vi "Startup.vi"(6 "LabVIEW Web Service":refnum<class "Web Service.lvclass">) -> ()   [LabVIEW 2014]
uses:
  <vilib>/wsapi/Web Service.lvclass
  DataManager/StateStore/Controls/DataFunction.ctl
panel:
  out "Array":cluster{"uuid":string, "int":i32}[](array[cluster])
  out "data out 2":string
  out "timing get SW 2":u32
  out "timing post SW 2":u32
  out "timing get 3":u32
  out "sum 2":i32
  out "timing post 2":u32
  out "timing get SW":u32
  out "timing post SW":u32
  out "timing post 1":u32
  out "data out":string
  out "service stopping?":bool
  out "timing get 2":u32
  out "sum":i32
  # "Use the web service input terminal to call the VIs on the Service subpalette of the Web Services palette. Do not remove it from the connector pane unless you don't need access to the palette."
  # "Any additional terminals added to the connector pane of a startup VI will be ignored."
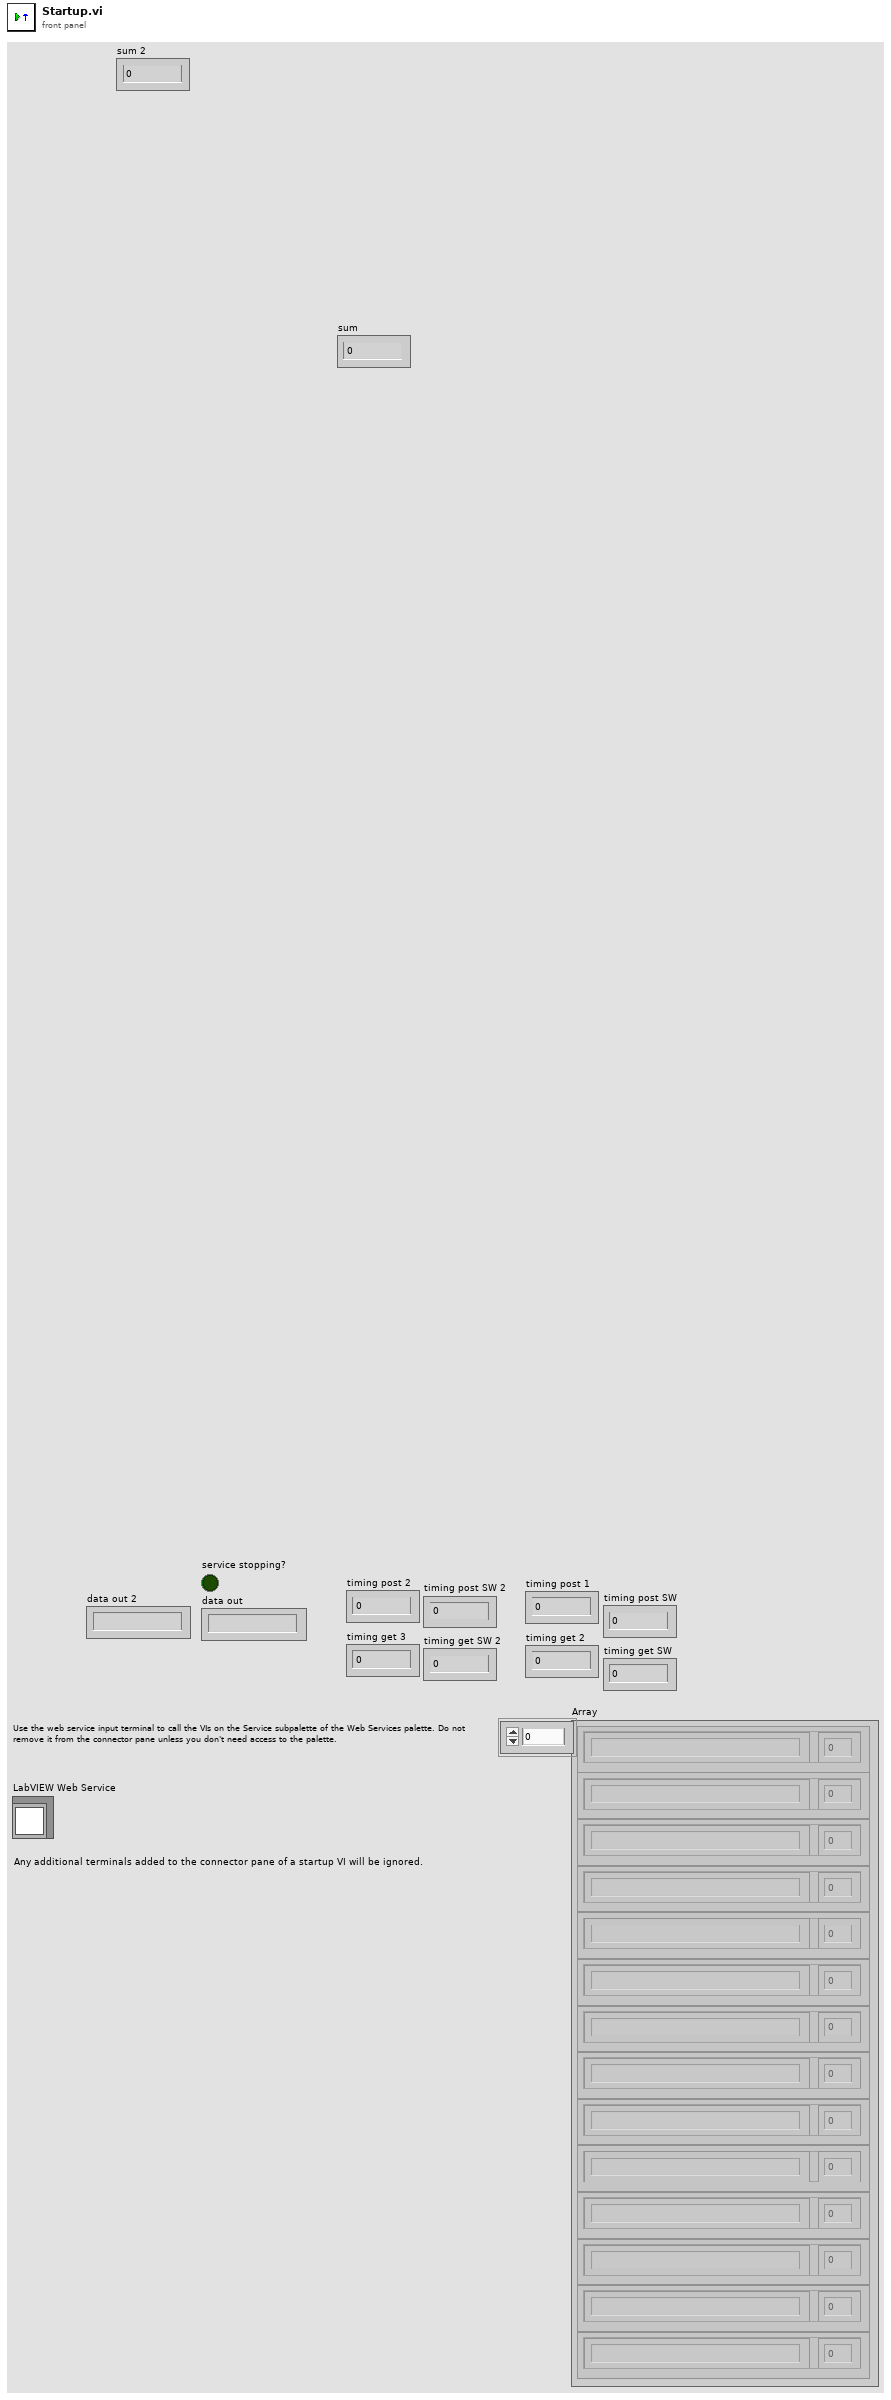
[diagram p1: front panel]
types:
  T1 = typedef "DataFunction.ctl" = enum16{"Initialise", "Release", "Get Data", "Set Data", "Preview Data"}
  T2 = enum16{"Standard", "Buffered", "CRLF", "Immediate"}
  T3 = cluster{"uuid":string, "int":i32, "posit_array":cluster{"x":dbl, "y":dbl, "z":dbl}[]}[]
  T4 = cluster{"0":string, "1":dbl, "2":dbl, "3":dbl, "4":dbl, "5":string, "6":string, "7":string}
  T5 = cluster{"switch_posit":cluster{"x":dbl, "y":dbl, "z":dbl}, "manual":bool}
  T6 = typedef "CData Core Control.ctl" = cluster{"train_data_array":cluster{"uuid":string, "int":i32, "posit_array":cluster{"x":dbl, "y":dbl, "z":dbl}[]}[], "train_control_array":cluster{"uuid":string, "throttle":dbl, "brake":dbl, "horn":dbl, "wait":dbl, "name":string, "mode":string, "dest":string}[], "switch_data_array":cluster{"switch_posit":cluster{"x":dbl, "y":dbl, "z":dbl}, "manual":bool}[], "switch_control_array":cluster{"switch_posit":cluster{"x":dbl, "y":dbl, "z":dbl}, "switch":bool, "invert":bool, "wait":dbl}[]}
  T7 = cluster{"uuid":string, "throttle":dbl, "brake":dbl, "horn":dbl, "wait":dbl, "name":string, "mode":string, "dest":string}[]
  T8 = cluster{"switch_posit":cluster{"x":dbl, "y":dbl, "z":dbl}, "manual":bool}[]
  T9 = cluster{"switch_posit":cluster{"x":dbl, "y":dbl, "z":dbl}, "switch":bool, "invert":bool, "wait":dbl}
  T10 = cluster{"switch_posit":cluster{"x":dbl, "y":dbl, "z":dbl}, "switch":bool, "invert":bool, "wait":dbl}[]
  T11 = cluster{"switch_posit":cluster{"x":dbl, "y":dbl, "z":dbl}, "switch":bool}
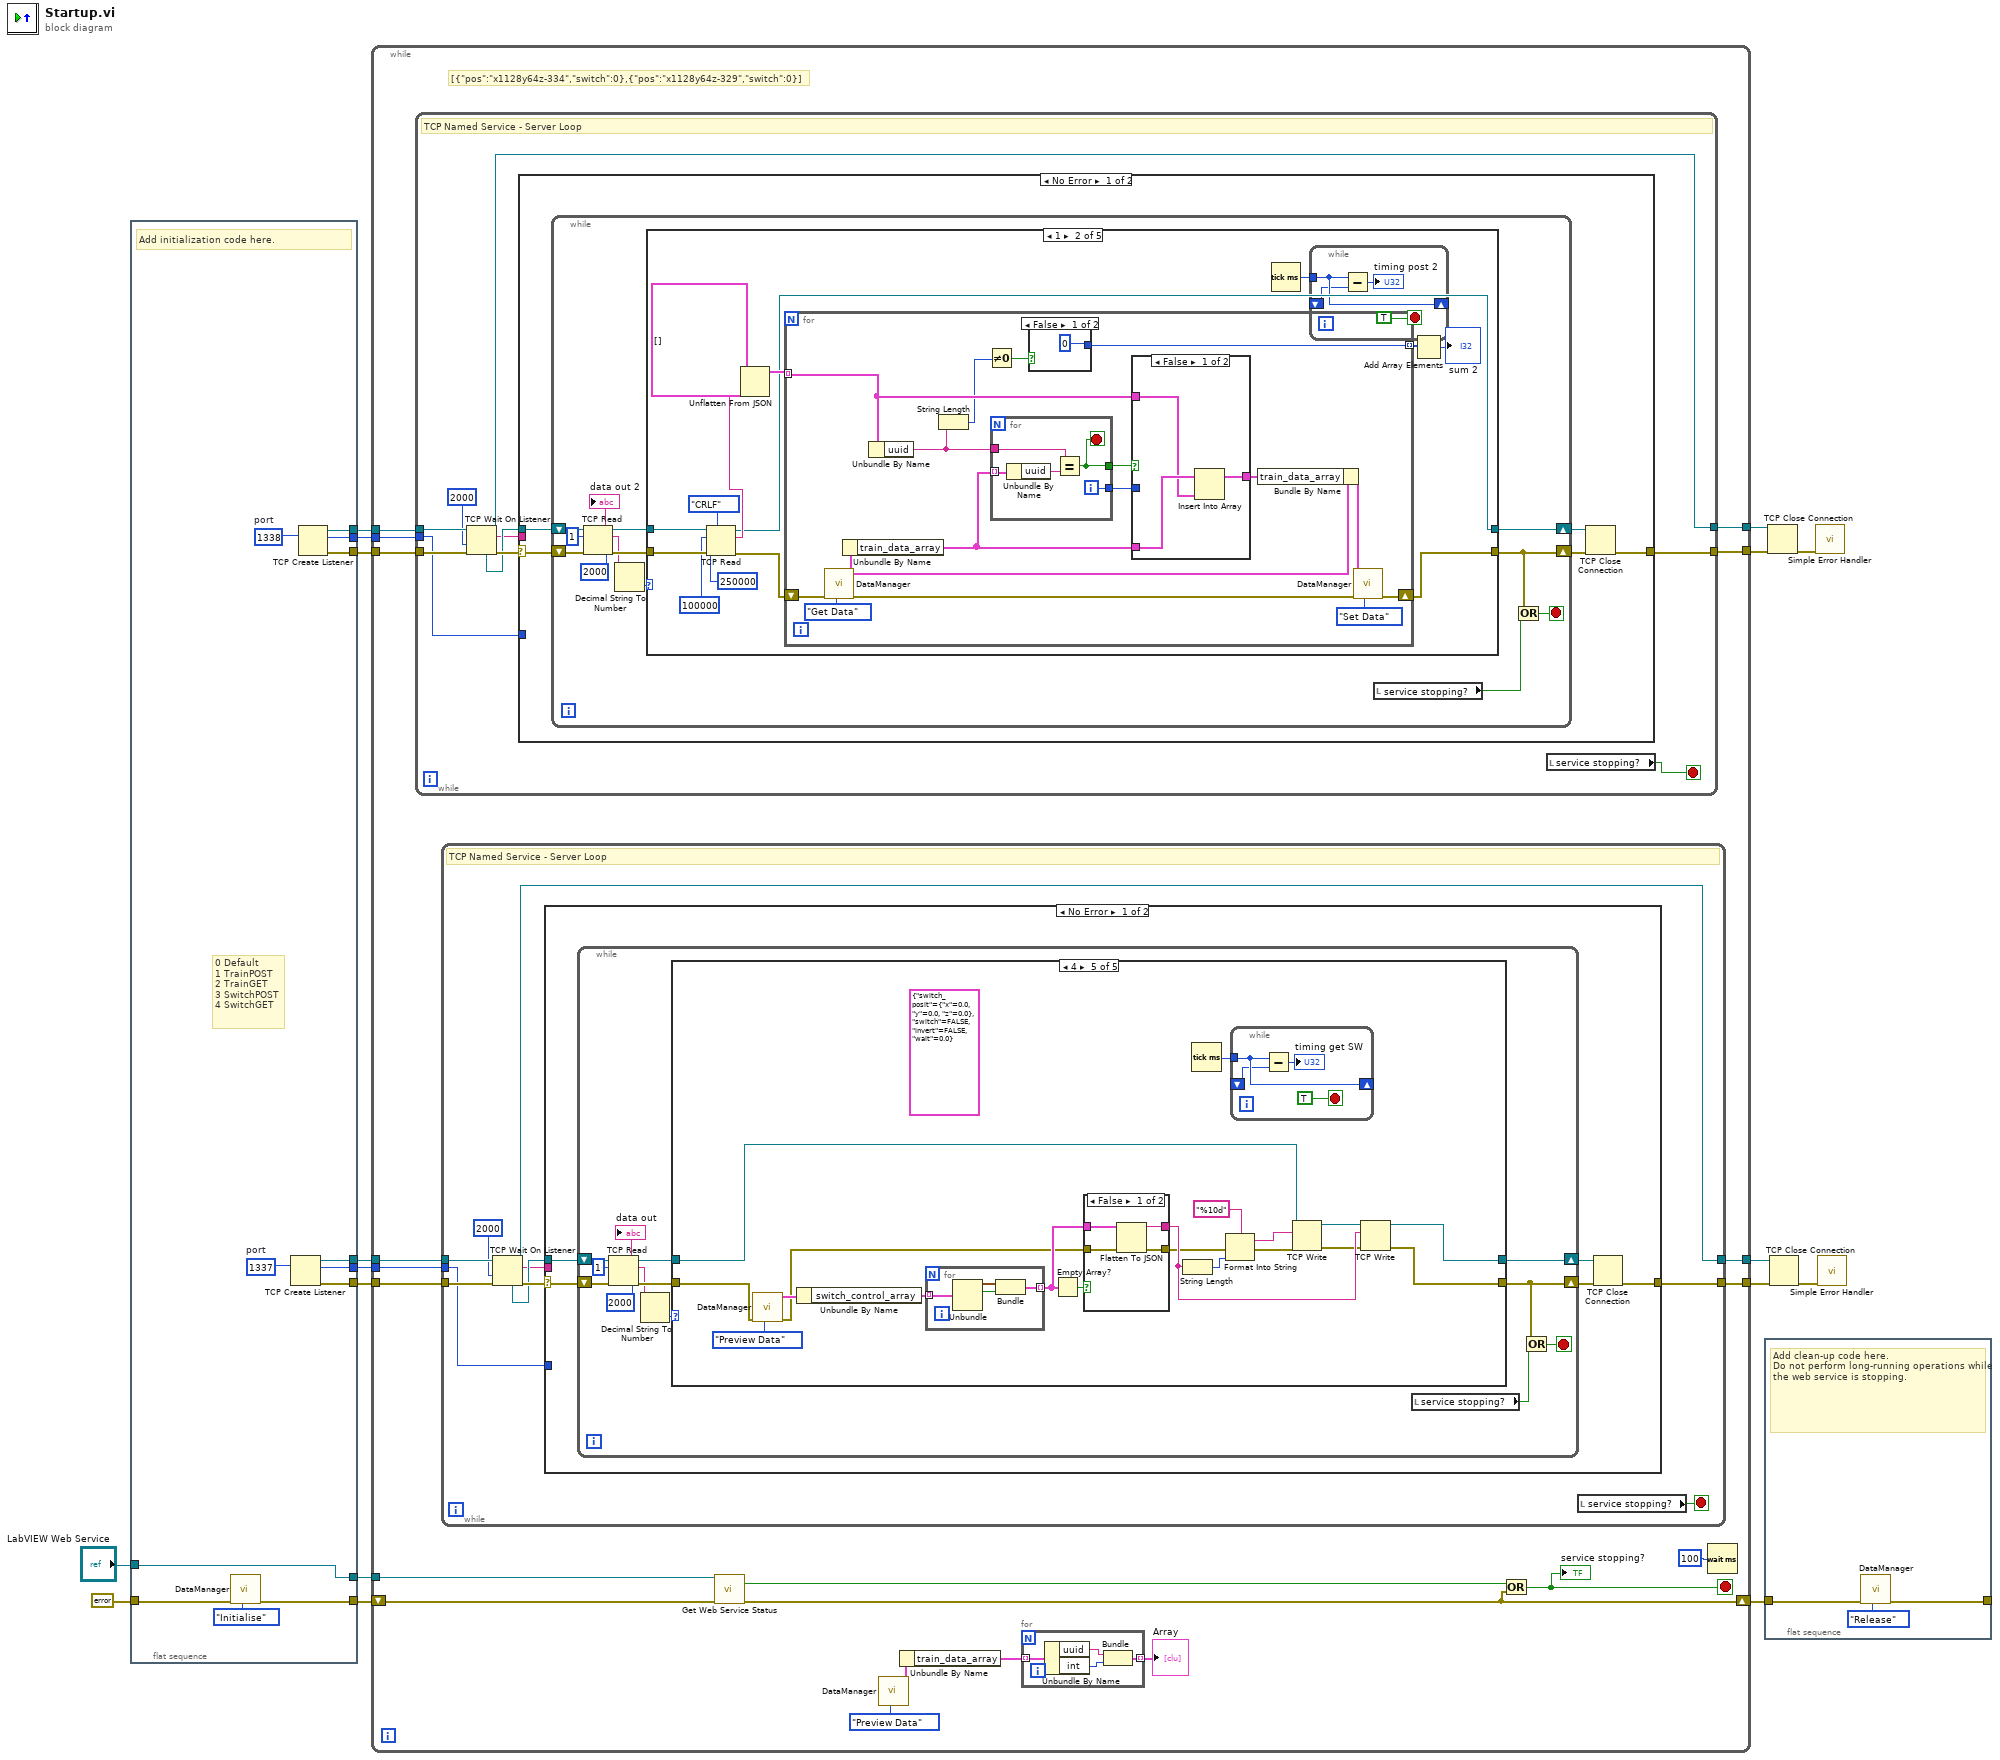
[diagram p0: block diagram]
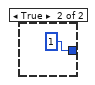
[diagram p3: hidden frame]
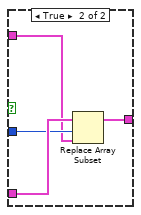
[diagram p4: hidden frame]
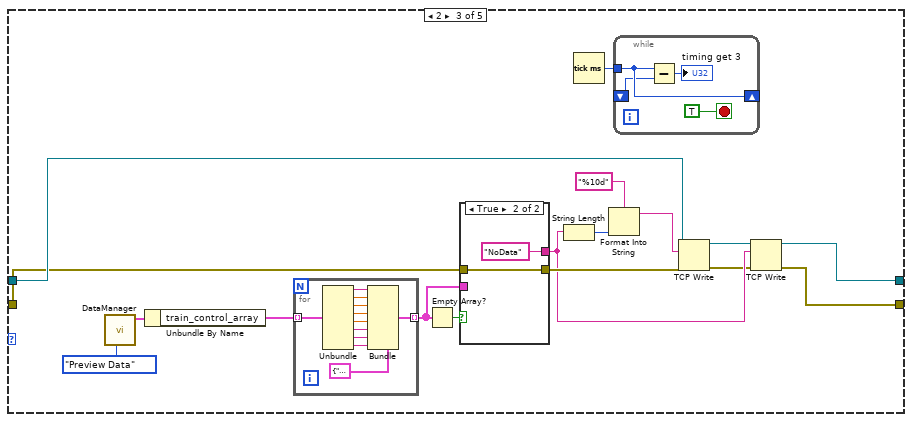
[diagram p5: hidden frame]
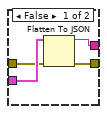
[diagram p6: hidden frame]
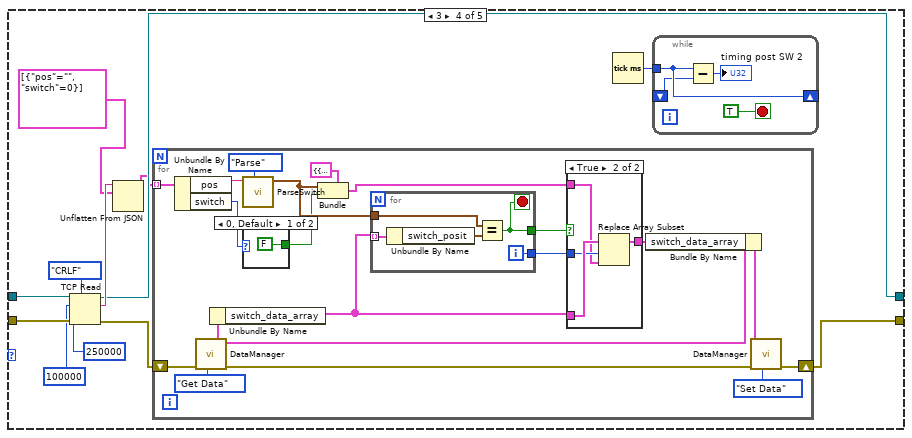
[diagram p7: hidden frame]
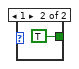
[diagram p8: hidden frame]
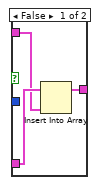
[diagram p9: hidden frame]
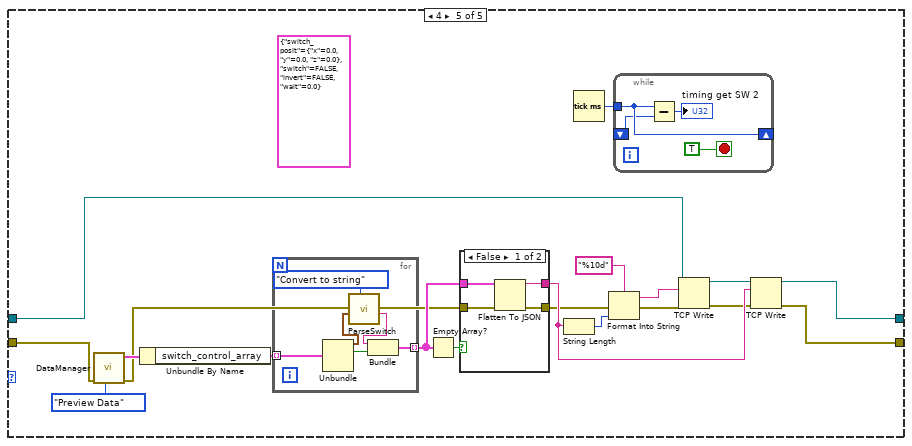
[diagram p10: hidden frame]
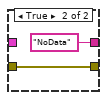
[diagram p11: hidden frame]
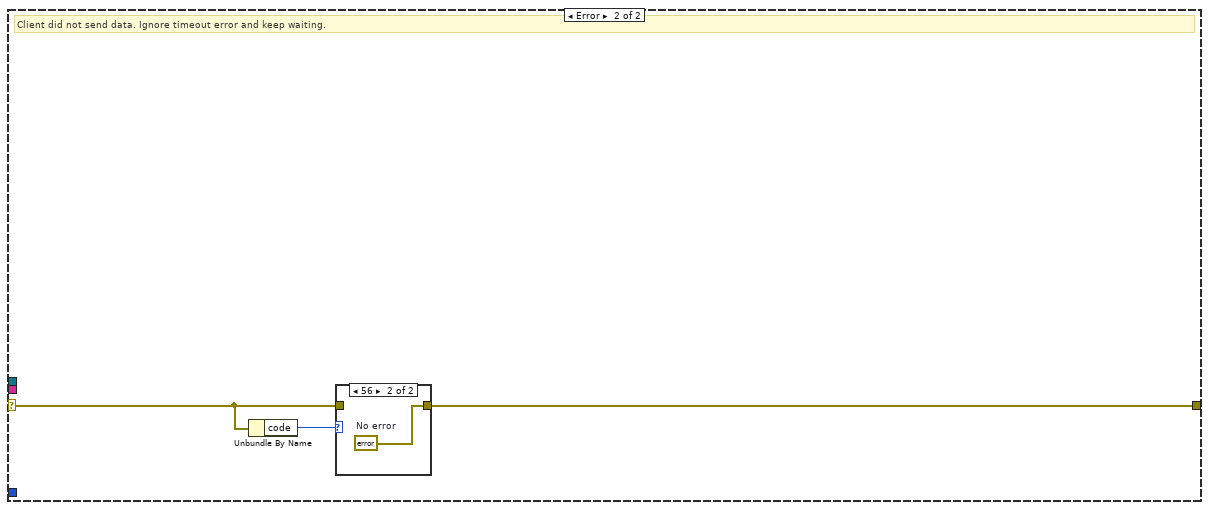
[diagram p12: hidden frame]
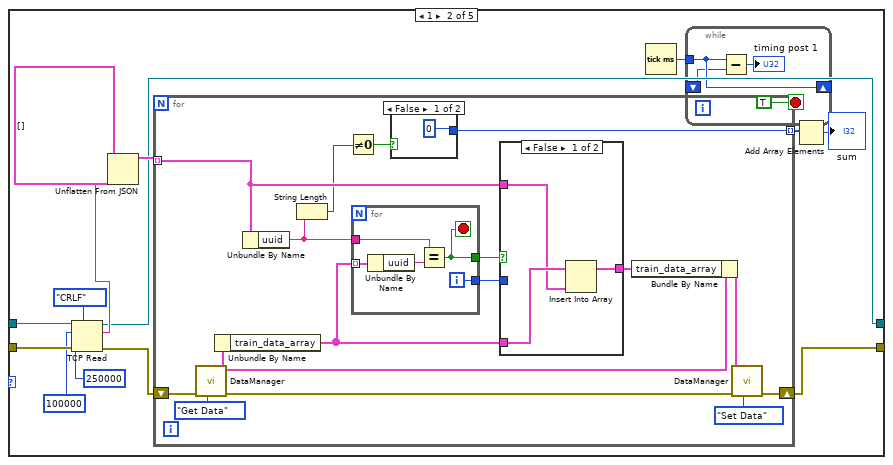
[diagram p15: hidden frame]
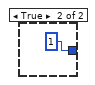
[diagram p16: hidden frame]
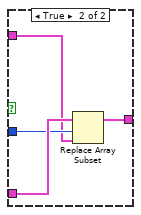
[diagram p17: hidden frame]
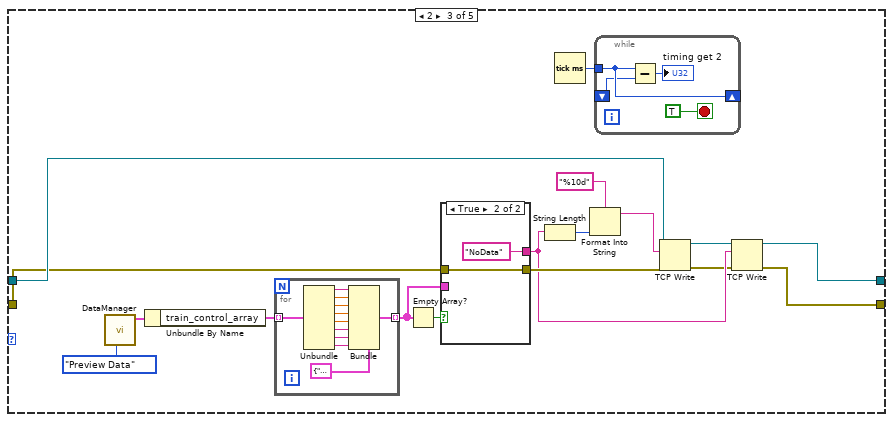
[diagram p18: hidden frame]
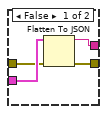
[diagram p19: hidden frame]
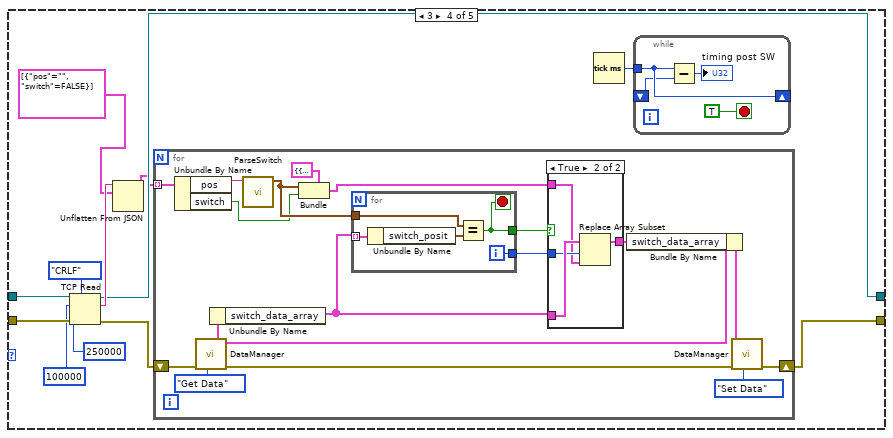
[diagram p20: hidden frame]
diagram:
  # "0 Default\n1 TrainPOST\n2 TrainGET\n3 SwitchPOST\n4 SwitchGET"
  n1 = flat-sequence {
    tunnel: "LabVIEW Web Service" -> [w29]
    tunnel: [w29] -> w16
    tunnel: [w18] -> w15
    tunnel: errorcluster {"status"=FALSE, "code"=0, "source"=""} ("error constant") -> [w19]
    tunnel: [w27] -> w9
    tunnel: [w26] -> w8
    tunnel: [w25] -> w7
    tunnel: [w23] -> w3
    tunnel: [w22] -> w2
    tunnel: [w21] -> w1
    frame #0 {
      w24 = u16 1338  # port
      w28 = u16 1337  # port
      # "Add initialization code here."
      n2 = call "DataManager.vi"("DataFunction"=DataFunction."Initialise", "error in (no error)"=w19) -> ("error out"=w18:errorcluster)  [unwired: 8 in, 1 out]
      n3 = TCP Create Listener(10:w28) -> (0:w25:errorcluster, 2:w26:u16, 3:w27:refnum<k5>)  [unwired: 4 in]
      n4 = TCP Create Listener(10:w24) -> (0:w22:errorcluster, 2:w21:u16, 3:w23:refnum<k5>)  [unwired: 4 in]
    }
  }
  n5 = while {
    tunnel: w16 -> [w48]
    shift-right: [w46] -> w13
    shift-left: w15 -> [w47]
    tunnel: [w44] -> w11
    tunnel: [w43] -> w10
    tunnel: w9 -> [w42]
    tunnel: w8 -> [w41]
    tunnel: w7 -> [w40]
    tunnel: [w38] -> w5
    tunnel: [w37] -> w4
    tunnel: w3 -> [w36]
    tunnel: w2 -> [w35]
    tunnel: w1 -> [w34]
    stop <- w39 stop-if-true
    # "[{\"pos\":\"x1128y64z-334\",\"switch\":0},{\"pos\":\"x1128y64z-329\",\"switch\":0}]"
    n6 = while {
      tunnel: [w55] -> w37
      tunnel: w36 -> [w63]
      tunnel: w35 -> [w61]
      tunnel: [w56] -> w38
      tunnel: w34 -> [w59]
      stop <- w54 stop-if-true
      # "TCP Named Service - Server Loop"
      n7 = TCP Wait On Listener(8:w61, 9:2000 ("timeout ms (25000)"), 11:w63) -> (0:w62:errorcluster, 2:w57:string, 3:w56:refnum<k5>, 4:w60:refnum<k5>)  [unwired: 1 in, 1 out]
      n8 = case shown="No Error" w62 {
        selector: w62 -> [w68 w255]
        tunnel: [w64 w253] -> w55
        tunnel: w60 -> [w67 _]
        tunnel: w59 -> [_ _]
        tunnel: w57 -> [_ _]
        frame No Error {
          n9 = while {
            shift-right: [w72] -> w65
            shift-left: w68 -> [w80]
            shift-right: [w70] -> w66
            shift-left: w67 -> [w79]
            stop <- w71 stop-if-true
            n10 = TCP Read(connection ID=w79, bytes to read=1, error in (no error)=w80, 9:2000 ("timeout ms (25000)")) -> (connection ID out=w75:refnum<k5>, data out=w74:string, error out=w76:errorcluster)  [unwired: 1 in]
            "data out 2" <- w74
            n11 = Decimal String To Number(string=w74) -> (number=w73:i32)  [unwired: 2 in, 1 out]
            n12 = case shown="1" w73 {
              tunnel: [w82 w86 w135 w174 w226] -> w72
              tunnel: w76 -> [w82 w92 w146 w180 w219]
              tunnel: w75 -> [w81 w91 w147 w179 w236]
              tunnel: [w81 w84 w134 w172 w225] -> w70
              frame 0, Default {
              }
              frame 1 {
                n13 = TCP Read(connection ID=w91, bytes to read=100000, error in (no error)=w92, 7:T2."CRLF" ("mode (standard)"), 9:250000 ("timeout ms (25000)")) -> (connection ID out=w84:refnum<k5>, data out=w90:string, error out=w85:errorcluster)
                n14 = Unflatten From JSON(JSON string=w90, type and defaults=T3 []) -> (value=w94:T3)  [unwired: 5 in, 1 out]
                n15 = for {
                  shift-right: [w108] -> w86
                  shift-left: w85 -> [w106]
                  tunnel: w94 -> [w105] mode=indexing
                  tunnel: [w101] -> w96 mode=indexing
                  n16 = call "DataManager.vi"("DataFunction"=DataFunction."Get Data", "error in (no error)"=w106) -> ("error out"=w107:errorcluster, "CData Out"=w109:T6)  [unwired: 8 in]
                  n17 = Unbundle By Name(w109) -> ("train_data_array"=w111:T3)
                  n18 = Unbundle By Name(w105) -> ("uuid"=w104:string)
                  n19 = String Length(string=w104) -> (length=w103:i32)
                  n20 = Not Equal To 0?(x=w103) -> (x != 0?=w102:bool)
                  n21 = for {
                    tunnel: w111 -> [w130] mode=indexing
                    tunnel: w104 -> [w128]
                    tunnel: [w127] -> w113
                    tunnel: [w126] -> w112
                    i -> [w126]
                    stop <- w127 stop-if-true
                    n22 = Unbundle By Name(w130) -> ("uuid"=w129:string)
                    n23 = Equal?(x=w128, y=w129) -> (x = y?=w127:bool)
                  }
                  n24 = case shown="False" w102 {
                    tunnel: [0 ("length") 1 ("length")] -> w101
                    frame False {
                    }
                    frame True {
                    }
                  }
                  n25 = case shown="False" w113 {
                    tunnel: w112 -> [_ w124]
                    tunnel: w111 -> [w121 w125]
                    tunnel: w105 -> [w120 w123]
                    tunnel: [w119 w122] -> w110
                    frame False {
                      n26 = Insert Into Array(array=w121, new element=w120) -> (w119:T3)  [unwired: 1 in]
                    }
                    frame True {
                      n27 = Replace Array Subset(array=w125, new element=w123, index=w124) -> (w122:T3)
                    }
                  }
                  n28 = Bundle By Name(cluster=w109, "train_data_array"=w110) -> (w114:T6)
                  n29 = call "DataManager.vi"("DataFunction"=DataFunction."Set Data", "error in (no error)"=w107, "CData In"=w114) -> ("error out"=w108:errorcluster)  [unwired: 7 in, 1 out]
                }
                n30 = Tick Count (ms)() -> (millisecond timer value=w83:u32)
                n31 = while {
                  tunnel: w83 -> [w100]
                  shift-right: [w100] -> _
                  shift-left: _ -> [w99]
                  stop <- TRUE stop-if-true
                  n32 = Subtract(x=w100, y=w99) -> (x-y=→"timing post 2":u32)
                }
                n33 = Add Array Elements(numeric array=w96) -> (sum=→"sum 2":i32)
              }
              frame 2 {
                n34 = call "DataManager.vi"("DataFunction"=DataFunction."Preview Data") -> ("CData Out"=w145:T6)  [unwired: 9 in, 1 out]
                n35 = Unbundle By Name(w145) -> ("train_control_array"=w143:T7)
                n36 = for {
                  tunnel: w143 -> [w168] mode=indexing
                  tunnel: [w159] -> w142 mode=indexing
                  n37 = Unbundle(w168) -> ("uuid"=w160:string, "throttle"=w161:dbl, "brake"=w162:dbl, "horn"=w163:dbl, "wait"=w164:dbl, "name"=w165:string, "mode"=w166:string, "dest"=w167:string)
                  n38 = Bundle(cluster=T4 {"0"="", "1"=0.0, "2"=0.0, "3"=0.0, "4"=0.0, "5"="", "6"="", "7"=""} ("train_control"), "0"=w160, "1"=w161, "2"=w162, "3"=w163, "4"=w164, "5"=w165, "6"=w166, "7"=w167) -> (w159:T4)
                }
                n39 = Empty Array?(array=w142) -> (empty?=w141:bool)
                n40 = case shown="True" w141 {
                  tunnel: [w155 "NoData" ("JSON string")] -> w137
                  tunnel: w142 -> [w154 _]
                  tunnel: w146 -> [w153 w157]
                  tunnel: [w152 w157] -> w140
                  frame False {
                    n41 = Flatten To JSON(anything=w154, error in (no error)=w153) -> (JSON string=w155:string, 11:w152:errorcluster)  [unwired: 1 in]
                  }
                  frame True {
                  }
                }
                n42 = String Length(string=w137) -> (length=w139:i32)
                n43 = Tick Count (ms)() -> (millisecond timer value=w131:u32)
                n44 = Format Into String(format string="%10d", w139) -> (resulting string=w132:string)  [unwired: 2 in, 1 out]
                n45 = while {
                  tunnel: w131 -> [w151]
                  shift-right: [w151] -> _
                  shift-left: _ -> [w150]
                  stop <- TRUE stop-if-true
                  n46 = Subtract(x=w151, y=w150) -> (x-y=→"timing get 3":u32)
                }
                n47 = TCP Write(connection ID=w147, data in=w132, error in (no error)=w140) -> (connection ID out=w133:refnum<k5>, error out=w136:errorcluster)  [unwired: 1 in, 1 out]
                n48 = TCP Write(connection ID=w133, data in=w137, error in (no error)=w136) -> (connection ID out=w134:refnum<k5>, error out=w135:errorcluster)  [unwired: 1 in, 1 out]
              }
              frame 3 {
                n49 = TCP Read(connection ID=w179, bytes to read=100000, error in (no error)=w180, 7:T2."CRLF" ("mode (standard)"), 9:250000 ("timeout ms (25000)")) -> (connection ID out=w172:refnum<k5>, data out=w178:string, error out=w173:errorcluster)
                n50 = Unflatten From JSON(JSON string=w178, type and defaults=cluster{"pos":string, "switch":i32}[] [{"pos"="", "switch"=0}]) -> (value=w169:cluster{"pos":string, "switch":i32}[])  [unwired: 5 in, 1 out]
                n51 = for {
                  shift-right: [w196] -> w174
                  shift-left: w173 -> [w194]
                  tunnel: w169 -> [w193] mode=indexing
                  n52 = Unbundle By Name(w193) -> ("pos"=w192:string, "switch"=w186:i32)
                  n53 = call "DataManager.vi"("DataFunction"=DataFunction."Get Data", "error in (no error)"=w194) -> ("error out"=w195:errorcluster, "CData Out"=w197:T6)  [unwired: 8 in]
                  n54 = Unbundle By Name(w197) -> ("switch_data_array"=w191:T8)
                  n55 = call "ParseSwitch.vi"("Enum"=enum16{"Parse", "Convert to string"}."Parse", "String"=w192) -> ("output cluster"=w189:cluster{"x":dbl, "y":dbl, "z":dbl})  [unwired: 8 in, 1 out]
                  n56 = case shown="0, Default" w186 {
                    tunnel: [FALSE ("manual") TRUE ("manual")] -> w185
                    frame 0, Default {
                    }
                    frame 1 {
                    }
                  }
                  n57 = Bundle(cluster=T5 {"switch_posit"={"x"=0.0, "y"=0.0, "z"=0.0}, "manual"=FALSE} ("new element/subarray"), "switch_posit"=w189, "manual"=w185) -> (w188:T5)
                  n58 = for {
                    tunnel: w191 -> [w217] mode=indexing
                    tunnel: [w215] -> w200
                    tunnel: [w214] -> w199
                    tunnel: w189 -> [w213]
                    i -> [w214]
                    stop <- w215 stop-if-true
                    n59 = Unbundle By Name(w217) -> ("switch_posit"=w216:cluster{"x":dbl, "y":dbl, "z":dbl})
                    n60 = Equal?(x=w213, y=w216) -> (x = y?=w215:bool)
                  }
                  n61 = case shown="True" w200 {
                    tunnel: w199 -> [_ w211]
                    tunnel: w191 -> [w208 w212]
                    tunnel: w188 -> [w207 w209]
                    tunnel: [w206 w210] -> w198
                    frame False {
                      n62 = Insert Into Array(array=w208, new element=w207) -> (w206:T8)  [unwired: 1 in]
                    }
                    frame True {
                      n63 = Replace Array Subset(array=w212, new element=w209, index=w211) -> (w210:T8)
                    }
                  }
                  n64 = Bundle By Name(cluster=w197, "switch_data_array"=w198) -> (w201:T6)
                  n65 = call "DataManager.vi"("DataFunction"=DataFunction."Set Data", "error in (no error)"=w195, "CData In"=w201) -> ("error out"=w196:errorcluster)  [unwired: 7 in, 1 out]
                }
                n66 = Tick Count (ms)() -> (millisecond timer value=w171:u32)
                n67 = while {
                  tunnel: w171 -> [w184]
                  shift-right: [w184] -> _
                  shift-left: _ -> [w183]
                  stop <- TRUE stop-if-true
                  n68 = Subtract(x=w184, y=w183) -> (x-y=→"timing post SW 2":u32)
                }
              }
              frame 4 {
                (unwired) T9 {"switch_posit"={"x"=0.0, "y"=0.0, "z"=0.0}, "switch"=FALSE, "invert"=FALSE, "wait"=0.0} ("switch_control")
                n69 = call "DataManager.vi"("DataFunction"=DataFunction."Preview Data", "error in (no error)"=w219) -> ("error out"=w218:errorcluster, "CData Out"=w235:T6)  [unwired: 8 in]
                n70 = Unbundle By Name(w235) -> ("switch_control_array"=w233:T10)
                n71 = for {
                  tunnel: w233 -> [w252] mode=indexing
                  tunnel: [w250] -> w232 mode=indexing
                  n72 = Unbundle(w252) -> ("switch_posit"=w248:cluster{"x":dbl, "y":dbl, "z":dbl}, "switch"=w251:bool)  [unwired: 2 out]
                  n73 = call "ParseSwitch.vi"("Enum"=enum16{"Parse", "Convert to string"}."Convert to string", "cluster in"=w248) -> ("pos"=w247:string)  [unwired: 8 in, 1 out]
                  n74 = Bundle("pos"=w247, "switch"=w251) -> (w250:cluster{"pos":string, "switch":bool})  [unwired: 1 in]
                }
                n75 = Empty Array?(array=w232) -> (empty?=w231:bool)
                n76 = case shown="False" w231 {
                  tunnel: [w244 "NoData" ("JSON string")] -> w228
                  tunnel: w232 -> [w243 _]
                  tunnel: w218 -> [w242 w246]
                  tunnel: [w241 w246] -> w221
                  frame False {
                    n77 = Flatten To JSON(anything=w243, error in (no error)=w242) -> (JSON string=w244:string, 11:w241:errorcluster)  [unwired: 1 in]
                  }
                  frame True {
                  }
                }
                n78 = String Length(string=w228) -> (length=w230:i32)
                n79 = Tick Count (ms)() -> (millisecond timer value=w222:u32)
                n80 = Format Into String(format string="%10d", error in=w221, w230) -> (resulting string=w223:string, error out=w220:errorcluster)  [unwired: 1 in]
                n81 = while {
                  tunnel: w222 -> [w240]
                  shift-right: [w240] -> _
                  shift-left: _ -> [w239]
                  stop <- TRUE stop-if-true
                  n82 = Subtract(x=w240, y=w239) -> (x-y=→"timing get SW 2":u32)
                }
                n83 = TCP Write(connection ID=w236, data in=w223, error in (no error)=w220) -> (connection ID out=w224:refnum<k5>, error out=w227:errorcluster)  [unwired: 1 in, 1 out]
                n84 = TCP Write(connection ID=w224, data in=w228, error in (no error)=w227) -> (connection ID out=w225:refnum<k5>, error out=w226:errorcluster)  [unwired: 1 in, 1 out]
              }
            }
            n85 = local read "service stopping?"() -> (w69:bool)
            n86 = Or(x=w72, y=w69) -> (x .or. y?=w71:bool)
          }
          n87 = TCP Close Connection(connection ID=w66, error in (no error)=w65) -> (error out=w64:errorcluster)  [unwired: 1 in, 1 out]
        }
        frame Error {
          # "Client did not send data. Ignore timeout error and keep waiting."
          n88 = Unbundle By Name(w255) -> ("code"=w254:i32)
          n89 = case shown="56" w254 {
            tunnel: w255 -> [w256 _]
            tunnel: [w256 w257] -> w253
            frame Default {
            }
            frame 56 {
              w257 = errorcluster {"status"=FALSE, "code"=0, "source"=""}  # No error
            }
          }
        }
      }
      n90 = local read "service stopping?"() -> (w54:bool)
    }
    n91 = while {
      tunnel: [w259] -> w43
      tunnel: w42 -> [w267]
      tunnel: w40 -> [w265]
      tunnel: [w260] -> w44
      tunnel: w41 -> [w263]
      stop <- w258 stop-if-true
      # "TCP Named Service - Server Loop"
      n92 = TCP Wait On Listener(8:w265, 9:2000 ("timeout ms (25000)"), 11:w267) -> (0:w266:errorcluster, 2:w261:string, 3:w260:refnum<k5>, 4:w264:refnum<k5>)  [unwired: 1 in, 1 out]
      n93 = case shown="No Error" w266 {
        selector: w266 -> [w272 w453]
        tunnel: [w268 w451] -> w259
        tunnel: w264 -> [w271 _]
        tunnel: w263 -> [_ _]
        tunnel: w261 -> [_ _]
        frame No Error {
          n94 = while {
            shift-right: [w276] -> w269
            shift-left: w272 -> [w284]
            shift-right: [w273] -> w270
            shift-left: w271 -> [w283]
            stop <- w274 stop-if-true
            n95 = TCP Read(connection ID=w283, bytes to read=1, error in (no error)=w284, 9:2000 ("timeout ms (25000)")) -> (connection ID out=w279:refnum<k5>, data out=w278:string, error out=w280:errorcluster)  [unwired: 1 in]
            "data out" <- w278
            n96 = Decimal String To Number(string=w278) -> (number=w277:i32)  [unwired: 2 in, 1 out]
            n97 = case shown="4" w277 {
              tunnel: [w286 w290 w339 w378 w426] -> w276
              tunnel: w280 -> [w286 w296 w350 w384 w419]
              tunnel: w279 -> [w285 w295 w351 w383 w436]
              tunnel: [w285 w288 w338 w376 w425] -> w273
              frame 0, Default {
              }
              frame 1 {
                n98 = TCP Read(connection ID=w295, bytes to read=100000, error in (no error)=w296, 7:T2."CRLF" ("mode (standard)"), 9:250000 ("timeout ms (25000)")) -> (connection ID out=w288:refnum<k5>, data out=w294:string, error out=w289:errorcluster)
                n99 = Unflatten From JSON(JSON string=w294, type and defaults=T3 []) -> (value=w298:T3)  [unwired: 5 in, 1 out]
                n100 = for {
                  shift-right: [w312] -> w290
                  shift-left: w289 -> [w310]
                  tunnel: w298 -> [w309] mode=indexing
                  tunnel: [w305] -> w300 mode=indexing
                  n101 = call "DataManager.vi"("DataFunction"=DataFunction."Get Data", "error in (no error)"=w310) -> ("error out"=w311:errorcluster, "CData Out"=w313:T6)  [unwired: 8 in]
                  n102 = Unbundle By Name(w313) -> ("train_data_array"=w315:T3)
                  n103 = Unbundle By Name(w309) -> ("uuid"=w308:string)
                  n104 = String Length(string=w308) -> (length=w307:i32)
                  n105 = Not Equal To 0?(x=w307) -> (x != 0?=w306:bool)
                  n106 = for {
                    tunnel: w315 -> [w334] mode=indexing
                    tunnel: w308 -> [w332]
                    tunnel: [w331] -> w317
                    tunnel: [w330] -> w316
                    i -> [w330]
                    stop <- w331 stop-if-true
                    n107 = Unbundle By Name(w334) -> ("uuid"=w333:string)
                    n108 = Equal?(x=w332, y=w333) -> (x = y?=w331:bool)
                  }
                  n109 = case shown="False" w306 {
                    tunnel: [0 ("length") 1 ("length")] -> w305
                    frame False {
                    }
                    frame True {
                    }
                  }
                  n110 = case shown="False" w317 {
                    tunnel: w316 -> [_ w328]
                    tunnel: w315 -> [w325 w329]
                    tunnel: w309 -> [w324 w327]
                    tunnel: [w323 w326] -> w314
                    frame False {
                      n111 = Insert Into Array(array=w325, new element=w324) -> (w323:T3)  [unwired: 1 in]
                    }
                    frame True {
                      n112 = Replace Array Subset(array=w329, new element=w327, index=w328) -> (w326:T3)
                    }
                  }
                  n113 = Bundle By Name(cluster=w313, "train_data_array"=w314) -> (w318:T6)
                  n114 = call "DataManager.vi"("DataFunction"=DataFunction."Set Data", "error in (no error)"=w311, "CData In"=w318) -> ("error out"=w312:errorcluster)  [unwired: 7 in, 1 out]
                }
                n115 = Tick Count (ms)() -> (millisecond timer value=w287:u32)
                n116 = while {
                  tunnel: w287 -> [w304]
                  shift-right: [w304] -> _
                  shift-left: _ -> [w303]
                  stop <- TRUE stop-if-true
                  n117 = Subtract(x=w304, y=w303) -> (x-y=→"timing post 1":u32)
                }
                n118 = Add Array Elements(numeric array=w300) -> (sum=→"sum":i32)
              }
              frame 2 {
                n119 = call "DataManager.vi"("DataFunction"=DataFunction."Preview Data") -> ("CData Out"=w349:T6)  [unwired: 9 in, 1 out]
                n120 = Unbundle By Name(w349) -> ("train_control_array"=w347:T7)
                n121 = for {
                  tunnel: w347 -> [w372] mode=indexing
                  tunnel: [w363] -> w346 mode=indexing
                  n122 = Unbundle(w372) -> ("uuid"=w364:string, "throttle"=w365:dbl, "brake"=w366:dbl, "horn"=w367:dbl, "wait"=w368:dbl, "name"=w369:string, "mode"=w370:string, "dest"=w371:string)
                  n123 = Bundle(cluster=T4 {"0"="", "1"=0.0, "2"=0.0, "3"=0.0, "4"=0.0, "5"="", "6"="", "7"=""} ("train_control"), "0"=w364, "1"=w365, "2"=w366, "3"=w367, "4"=w368, "5"=w369, "6"=w370, "7"=w371) -> (w363:T4)
                }
                n124 = Empty Array?(array=w346) -> (empty?=w345:bool)
                n125 = case shown="True" w345 {
                  tunnel: [w359 "NoData" ("JSON string")] -> w341
                  tunnel: w346 -> [w358 _]
                  tunnel: w350 -> [w357 w361]
                  tunnel: [w356 w361] -> w344
                  frame False {
                    n126 = Flatten To JSON(anything=w358, error in (no error)=w357) -> (JSON string=w359:string, 11:w356:errorcluster)  [unwired: 1 in]
                  }
                  frame True {
                  }
                }
                n127 = String Length(string=w341) -> (length=w343:i32)
                n128 = Tick Count (ms)() -> (millisecond timer value=w335:u32)
                n129 = Format Into String(format string="%10d", w343) -> (resulting string=w336:string)  [unwired: 2 in, 1 out]
                n130 = while {
                  tunnel: w335 -> [w355]
                  shift-right: [w355] -> _
                  shift-left: _ -> [w354]
                  stop <- TRUE stop-if-true
                  n131 = Subtract(x=w355, y=w354) -> (x-y=→"timing get 2":u32)
                }
                n132 = TCP Write(connection ID=w351, data in=w336, error in (no error)=w344) -> (connection ID out=w337:refnum<k5>, error out=w340:errorcluster)  [unwired: 1 in, 1 out]
                n133 = TCP Write(connection ID=w337, data in=w341, error in (no error)=w340) -> (connection ID out=w338:refnum<k5>, error out=w339:errorcluster)  [unwired: 1 in, 1 out]
              }
              frame 3 {
                n134 = TCP Read(connection ID=w383, bytes to read=100000, error in (no error)=w384, 7:T2."CRLF" ("mode (standard)"), 9:250000 ("timeout ms (25000)")) -> (connection ID out=w376:refnum<k5>, data out=w382:string, error out=w377:errorcluster)
                n135 = Unflatten From JSON(JSON string=w382, type and defaults=cluster{"pos":string, "switch":bool}[] [{"pos"="", "switch"=FALSE}]) -> (value=w373:cluster{"pos":string, "switch":bool}[])  [unwired: 5 in, 1 out]
                n136 = for {
                  shift-right: [w398] -> w378
                  shift-left: w377 -> [w396]
                  tunnel: w373 -> [w395] mode=indexing
                  n137 = Unbundle By Name(w395) -> ("pos"=w394:string, "switch"=w390:bool)
                  n138 = call "DataManager.vi"("DataFunction"=DataFunction."Get Data", "error in (no error)"=w396) -> ("error out"=w397:errorcluster, "CData Out"=w399:T6)  [unwired: 8 in]
                  n139 = Unbundle By Name(w399) -> ("switch_data_array"=w393:T8)
                  n140 = call "ParseSwitch.vi"("String"=w394) -> ("output cluster"=w391:cluster{"x":dbl, "y":dbl, "z":dbl})  [unwired: 9 in, 1 out]
                  n141 = Bundle(cluster=T5 {"switch_posit"={"x"=0.0, "y"=0.0, "z"=0.0}, "manual"=FALSE} ("new element/subarray"), "switch_posit"=w391, "manual"=w390) -> (w389:T5)
                  n142 = for {
                    tunnel: w393 -> [w417] mode=indexing
                    tunnel: [w415] -> w402
                    tunnel: [w414] -> w401
                    tunnel: w391 -> [w413]
                    i -> [w414]
                    stop <- w415 stop-if-true
                    n143 = Unbundle By Name(w417) -> ("switch_posit"=w416:cluster{"x":dbl, "y":dbl, "z":dbl})
                    n144 = Equal?(x=w413, y=w416) -> (x = y?=w415:bool)
                  }
                  n145 = case shown="True" w402 {
                    tunnel: w401 -> [_ w411]
                    tunnel: w393 -> [w408 w412]
                    tunnel: w389 -> [w407 w409]
                    tunnel: [w406 w410] -> w400
                    frame False {
                      n146 = Insert Into Array(array=w408, new element=w407) -> (w406:T8)  [unwired: 1 in]
                    }
                    frame True {
                      n147 = Replace Array Subset(array=w412, new element=w409, index=w411) -> (w410:T8)
                    }
                  }
                  n148 = Bundle By Name(cluster=w399, "switch_data_array"=w400) -> (w403:T6)
                  n149 = call "DataManager.vi"("DataFunction"=DataFunction."Set Data", "error in (no error)"=w397, "CData In"=w403) -> ("error out"=w398:errorcluster)  [unwired: 7 in, 1 out]
                }
                n150 = Tick Count (ms)() -> (millisecond timer value=w375:u32)
                n151 = while {
                  tunnel: w375 -> [w388]
                  shift-right: [w388] -> _
                  shift-left: _ -> [w387]
                  stop <- TRUE stop-if-true
                  n152 = Subtract(x=w388, y=w387) -> (x-y=→"timing post SW":u32)
                }
              }
              frame 4 {
                (unwired) T9 {"switch_posit"={"x"=0.0, "y"=0.0, "z"=0.0}, "switch"=FALSE, "invert"=FALSE, "wait"=0.0} ("switch_control")
                n153 = call "DataManager.vi"("DataFunction"=DataFunction."Preview Data", "error in (no error)"=w419) -> ("error out"=w418:errorcluster, "CData Out"=w435:T6)  [unwired: 8 in]
                n154 = Unbundle By Name(w435) -> ("switch_control_array"=w433:T10)
                n155 = for {
                  tunnel: w433 -> [w450] mode=indexing
                  tunnel: [w447] -> w432 mode=indexing
                  n156 = Unbundle(w450) -> ("switch_posit"=w448:cluster{"x":dbl, "y":dbl, "z":dbl}, "switch"=w449:bool)  [unwired: 2 out]
                  n157 = Bundle("switch_posit"=w448, "switch"=w449) -> (w447:T11)  [unwired: 1 in]
                }
                n158 = Empty Array?(array=w432) -> (empty?=w431:bool)
                n159 = case shown="False" w431 {
                  tunnel: [w444 "NoData" ("JSON string")] -> w428
                  tunnel: w432 -> [w443 _]
                  tunnel: w418 -> [w442 w446]
                  tunnel: [w441 w446] -> w421
                  frame False {
                    n160 = Flatten To JSON(anything=w443, error in (no error)=w442) -> (JSON string=w444:string, 11:w441:errorcluster)  [unwired: 1 in]
                  }
                  frame True {
                  }
                }
                n161 = String Length(string=w428) -> (length=w430:i32)
                n162 = Tick Count (ms)() -> (millisecond timer value=w422:u32)
                n163 = Format Into String(format string="%10d", error in=w421, w430) -> (resulting string=w423:string, error out=w420:errorcluster)  [unwired: 1 in]
                n164 = while {
                  tunnel: w422 -> [w440]
                  shift-right: [w440] -> _
                  shift-left: _ -> [w439]
                  stop <- TRUE stop-if-true
                  n165 = Subtract(x=w440, y=w439) -> (x-y=→"timing get SW":u32)
                }
                n166 = TCP Write(connection ID=w436, data in=w423, error in (no error)=w420) -> (connection ID out=w424:refnum<k5>, error out=w427:errorcluster)  [unwired: 1 in, 1 out]
                n167 = TCP Write(connection ID=w424, data in=w428, error in (no error)=w427) -> (connection ID out=w425:refnum<k5>, error out=w426:errorcluster)  [unwired: 1 in, 1 out]
              }
            }
            n168 = local read "service stopping?"() -> (w275:bool)
            n169 = Or(x=w276, y=w275) -> (x .or. y?=w274:bool)
          }
          n170 = TCP Close Connection(connection ID=w270, error in (no error)=w269) -> (error out=w268:errorcluster)  [unwired: 1 in, 1 out]
        }
        frame Error {
          # "Client did not send data. Ignore timeout error and keep waiting."
          n171 = Unbundle By Name(w453) -> ("code"=w452:i32)
          n172 = case shown="56" w452 {
            tunnel: w453 -> [w454 _]
            tunnel: [w454 w455] -> w451
            frame Default {
            }
            frame 56 {
              w455 = errorcluster {"status"=FALSE, "code"=0, "source"=""}  # No error
            }
          }
        }
      }
      n173 = local read "service stopping?"() -> (w258:bool)
    }
    n174 = call <vilib>:"Get Web Service Status.vi"("LabVIEW Web Service"=w48, "error in (no error)"=w47) -> ("service stopping?"=w49:bool, "error out"=w46:errorcluster)  [unwired: 11 in, 1 out]
    n175 = call "DataManager.vi"("DataFunction"=DataFunction."Preview Data") -> ("CData Out"=w32:T6)  [unwired: 9 in, 1 out]
    n176 = Unbundle By Name(w32) -> ("train_data_array"=w31:T3)
    n177 = for {
      tunnel: w31 -> [w53] mode=indexing
      tunnel: [w50] -> w30 mode=indexing
      n178 = Unbundle By Name(w53) -> ("uuid"=w51:string, "int"=w52:i32)
      n179 = Bundle("uuid"=w51, "int"=w52) -> (w50:cluster{"uuid":string, "int":i32})  [unwired: 1 in]
    }
    "Array" <- w30
    n180 = Or(x=w49, y=w46) -> (x .or. y?=w39:bool)
    "service stopping?" <- w39
    n181 = Wait (ms)(milliseconds to wait=u32 100) -> ()  [unwired: 1 out]
  }
  n182 = flat-sequence {
    tunnel: w13 -> [w457]
    tunnel: [w456] -> _
    frame #0 {
      # "Add clean-up code here.\nDo not perform long-running operations while the web service is stopping."
      n183 = call "DataManager.vi"("DataFunction"=DataFunction."Release", "error in (no error)"=w457) -> ("error out"=w456:errorcluster)  [unwired: 8 in, 1 out]
    }
  }
  n184 = TCP Close Connection(connection ID=w5, error in (no error)=w4) -> (error out=w6:errorcluster)  [unwired: 1 in, 1 out]
  n185 = TCP Close Connection(connection ID=w11, error in (no error)=w10) -> (error out=w12:errorcluster)  [unwired: 1 in, 1 out]
  n186 = call <vilib>:"Simple Error Handler.vi"("error in (no error)"=w6) -> ()  [unwired: 4 in, 5 out]
  n187 = call <vilib>:"Simple Error Handler.vi"("error in (no error)"=w12) -> ()  [unwired: 4 in, 5 out]
